vi "Simulate_RV_Core.vi"() -> ()   [LabVIEW 2011]
doc: "I. Description:\nThis example demonstrates how to continuously output a waveform using an internal sample clock. The automatic regeneration of data has been disabled, so new data has to be provided throughout the duration of the continuous Analog Output operation. This allows the generation of any arbitrary frequency as this VI computes new data for each iteration of the loop, maintaining phase continuity of the signal.\n\nII. Instructions for Running:\n1. Select the Physical Channel to correspond to where your signal is output on the DAQ device.\n2. Enter the Minimum and Maximum Voltage range.\n3. Specify the desired Sample Clock Rate of the output Waveform. Higher sample clock rates will produce a smoother waveform.\n4. Manually specify the Analog Output buffer size, in number of samples. A larger buffer would help non-regenerative operations avoid errors due to occasional high CPU load. \nNote: \nThe Analog Output buffer has to be at least as big as the amount of data being written to the board per iteration. The recommended buffer size would be at least twice the amount of data being written to the board per iteration.\n5. Enter the Waveform Information. See the documentation of the Basic Function Generator SubVI for information on each parameter.\n\nIII. Block Diagram Steps:\n1. Create an Analog Output Voltage channel.\n2. Configure the task to prohibit the automatic regeneration of data.\n3. Call the DAQmx (Sample Clock) VI to set the sample clock rate. Additionally, set the sample mode to Continuous.\n4. Read the actual sample clock rate (eventually coerced depending on the hardware used). \n5. Compute the desired waveform, using the buffer size and the actual update rate. This VI keeps track of the phase of the waveform to ensure that the generated signal is continuous.\n6. Write the waveform to the output buffer. \n7a. Call the Start VI. This is only needed when the loop is executed for the first time.\n7b. Do nothing.\n8. Loop continuously until user presses the Stop button. Every iteration computes and writes a new waveform to the buffer.\n9. Call the Clear Task VI to clear the Task.\n10. Use the popup dialog box to display an error or warning if any.\n\nIV. I/O Connections Overview:\nMake sure your signal output terminal matches the Physical Channel I/O Control. For further connection information, refer to your hardware reference manual."
uses:
  <vilib>/Utility/error.llb/DialogType.ctl
  <vilib>/DAQmx/write.llb/DAQmx Write (Analog 1D Wfm NChan NSamp).vi
  <vilib>/DAQmx/create/channels.llb/DAQmx Create Channel (AO-Voltage-Basic).vi
  <vilib>/DAQmx/configure/timing.llb/DAQmx Timing (Sample Clock).vi
  <vilib>/DAQmx/miscellaneous.llb/DAQmx Fill In Error Info.vi
  <vilib>/measure/NI_MABase.lvlib
  Program Files (x86)/National Instruments/LabVIEW 2011/resource/objmgr/daqmx.rc
panel:
  in  "Tab Control":T1(tab)=enum."RV"
  out "Trigger":waveform(dbl)(graph)={"t0"=timestamp(78.0 s since 1904-01-01), "dt"=0.0006666666666666666, "Y"=array[1200 elements]}
  in  "Trigg. level":sgl=2.0
  in  "Regular level":sgl=10.0
  in  "RV009_Ph":sgl[](array[numeric])=[0.0, 0.0, 0.0]
  in  "RV009_Amp":sgl[](array[numeric])=[0.9, 0.0, 0.0]
  in  "RV009.DC":sgl=5.0
  in  "RV008_Ph":sgl[](array[numeric])=[0.0, 0.0, 0.0]
  in  "RV008_Amp":sgl[](array[numeric])=[0.8, 0.0, 0.0]
  in  "RV008.DC":sgl=5.0
  in  "RV007_Ph":sgl[](array[numeric])=[0.0, 0.0, 0.0]
  in  "RV007_Amp":sgl[](array[numeric])=[0.4, 0.3, 0.4]
  in  "RV007.DC":sgl=5.0
  in  "RV006_Ph":sgl[](array[numeric])=[0.0, 0.0, 0.0]
  in  "RV006_Amp":sgl[](array[numeric])=[0.7, 0.3, 0.5]
  in  "RV006.DC":sgl=5.0
  out "RV":waveform(dbl)[](graph)=[{"t0"=timestamp(78.0 s since 1904-01-01), "dt"=0.0006666666666666666, "Y"=array[1200 elements]}, {"t0"=timestamp(78.0 s since 1904-01-01), "dt"=0.0006666666666666666, "Y"=array[1200 elements]}, {"t0"=timestamp(78.0 s since 1904-01-01), "dt"=0.0006666666666666666, "Y"=array[1200 elements]}, {"t0"=timestamp(78.0 s since 1904-01-01), "dt"=0.0006666666666666666, "Y"=array[1200 elements]}, {"t0"=timestamp(78.0 s since 1904-01-01), "dt"=0.0006666666666666666, "Y"=array[1200 elements]}, {"t0"=timestamp(78.0 s since 1904-01-01), "dt"=0.0006666666666666666, "Y"=array[1200 elements]}, {"t0"=timestamp(78.0 s since 1904-01-01), "dt"=0.0006666666666666666, "Y"=array[1200 elements]}, {"t0"=timestamp(78.0 s since 1904-01-01), "dt"=0.0006666666666666666, "Y"=array[1200 elements]}, {"t0"=timestamp(78.0 s since 1904-01-01), "dt"=0.0006666666666666666, "Y"=array[1200 elements]}, {"t0"=timestamp(78.0 s since 1904-01-01), "dt"=0.0006666666666666666, "Y"=array[1200 elements]}]
  in  "RV000_Ph":sgl[](array[numeric])=[0.0, 0.0, 0.0]
  in  "RV000_Amp":sgl[](array[numeric])=[0.4, 0.1, 0.3]
  in  "RV000.DC":sgl=5.0
  in  "RV001.DC":sgl=5.0
  in  "RV001_Amp":sgl[](array[numeric])=[0.8, 0.6, 0.2]
  in  "RV001_Ph":sgl[](array[numeric])=[90.0, 0.0, 0.0]
  in  "RV002_Ph":sgl[](array[numeric])=[0.0, 0.0, 0.0]
  in  "RV002_Amp":sgl[](array[numeric])=[0.3, 0.5, 0.3]
  in  "RV002.DC":sgl=5.0
  in  "RV003_Ph":sgl[](array[numeric])=[90.0, 0.0, 0.0]
  in  "RV003_Amp":sgl[](array[numeric])=[0.7, 0.4, 0.2]
  in  "RV003.DC":sgl=5.0
  in  "Multiplication factor":dbl=0.5
  in  "Add Noise":bool
  in  "RV004_Ph":sgl[](array[numeric])=[0.0, 0.0, 0.0]
  in  "RV004_Amp":sgl[](array[numeric])=[0.6, 0.3, 0.1]
  in  "RV004.DC":sgl=5.0
  in  "RV005_Ph":sgl[](array[numeric])=[0.0, 0.0, 0.0]
  in  "RV005_Amp":sgl[](array[numeric])=[0.9, 0.4, 0.2]
  in  "RV005.DC":sgl=5.0
  out "Proc1":waveform(dbl)(graph)={"t0"=timestamp(78.0 s since 1904-01-01), "dt"=0.0006666666666666666, "Y"=array[1200 elements]}
  in  "DC Proc Val 1":sgl=6.0
  out "Proc2":waveform(dbl)(graph)={"t0"=timestamp(78.0 s since 1904-01-01), "dt"=0.0006666666666666666, "Y"=array[1200 elements]}
  in  "DC Proc Val 2":sgl=1.0
  out "Loop Iteration":dbl=0.8050460815429688
  out "Waveform Graph":waveform(dbl)[](graph)=[{"t0"=timestamp(78.0 s since 1904-01-01), "dt"=0.0006666666666666666, "Y"=array[1200 elements]}, {"t0"=timestamp(78.0 s since 1904-01-01), "dt"=0.0006666666666666666, "Y"=array[1200 elements]}, {"t0"=timestamp(78.0 s since 1904-01-01), "dt"=0.0006666666666666666, "Y"=array[1200 elements]}, {"t0"=timestamp(78.0 s since 1904-01-01), "dt"=0.0006666666666666666, "Y"=array[1200 elements]}, {"t0"=timestamp(78.0 s since 1904-01-01), "dt"=0.0006666666666666666, "Y"=array[1200 elements]}, {"t0"=timestamp(78.0 s since 1904-01-01), "dt"=0.0006666666666666666, "Y"=array[1200 elements]}, {"t0"=timestamp(78.0 s since 1904-01-01), "dt"=0.0006666666666666666, "Y"=array[1200 elements]}, {"t0"=timestamp(78.0 s since 1904-01-01), "dt"=0.0006666666666666666, "Y"=array[1200 elements]}, {"t0"=timestamp(78.0 s since 1904-01-01), "dt"=0.0006666666666666666, "Y"=array[1200 elements]}, {"t0"=timestamp(78.0 s since 1904-01-01), "dt"=0.0006666666666666666, "Y"=array[1200 elements]}, {"t0"=timestamp(78.0 s since 1904-01-01), "dt"=0.0006666666666666666, "Y"=array[1200 elements]}, {"t0"=timestamp(78.0 s since 1904-01-01), "dt"=0.0006666666666666666, "Y"=array[1200 elements]}, {"t0"=timestamp(78.0 s since 1904-01-01), "dt"=0.0006666666666666666, "Y"=array[1200 elements]}] caption="Output Waveforms"
  in  "stop":bool
  # "s"
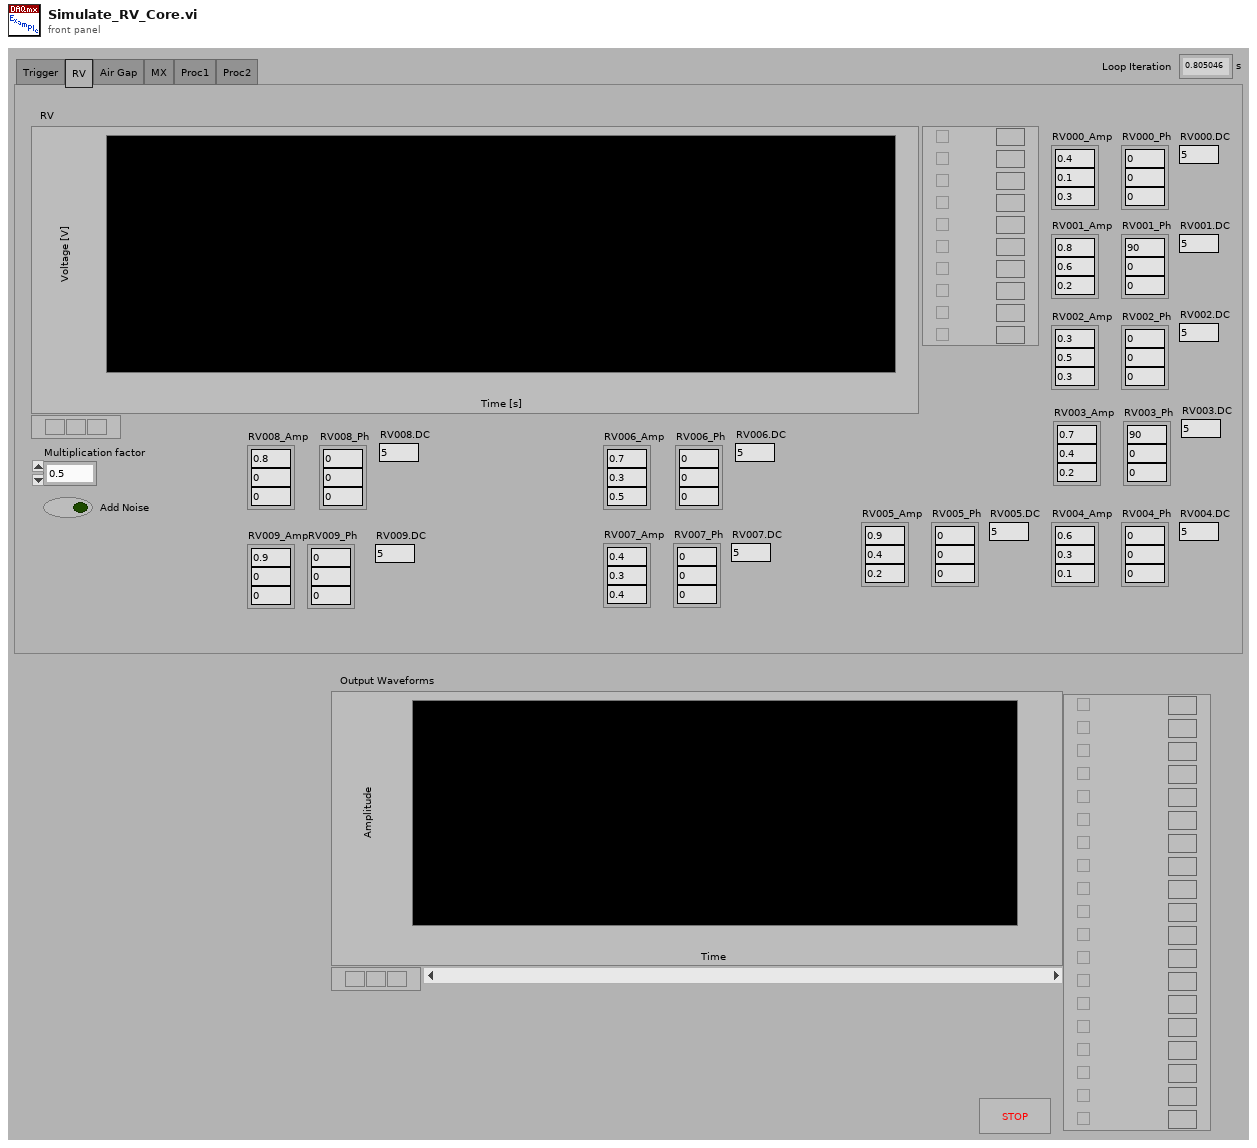
[diagram p1: front panel]
types:
  T1 = enum32{"Trigger", "RV", "Air Gap", "MX", "Proc1", "Proc2"}
  T2 = typedef "DialogType.ctl" = u16
  T3 = enum16{"Sine Wave", "Triangle Wave", "Square Wave", "Sawtooth Wave"}
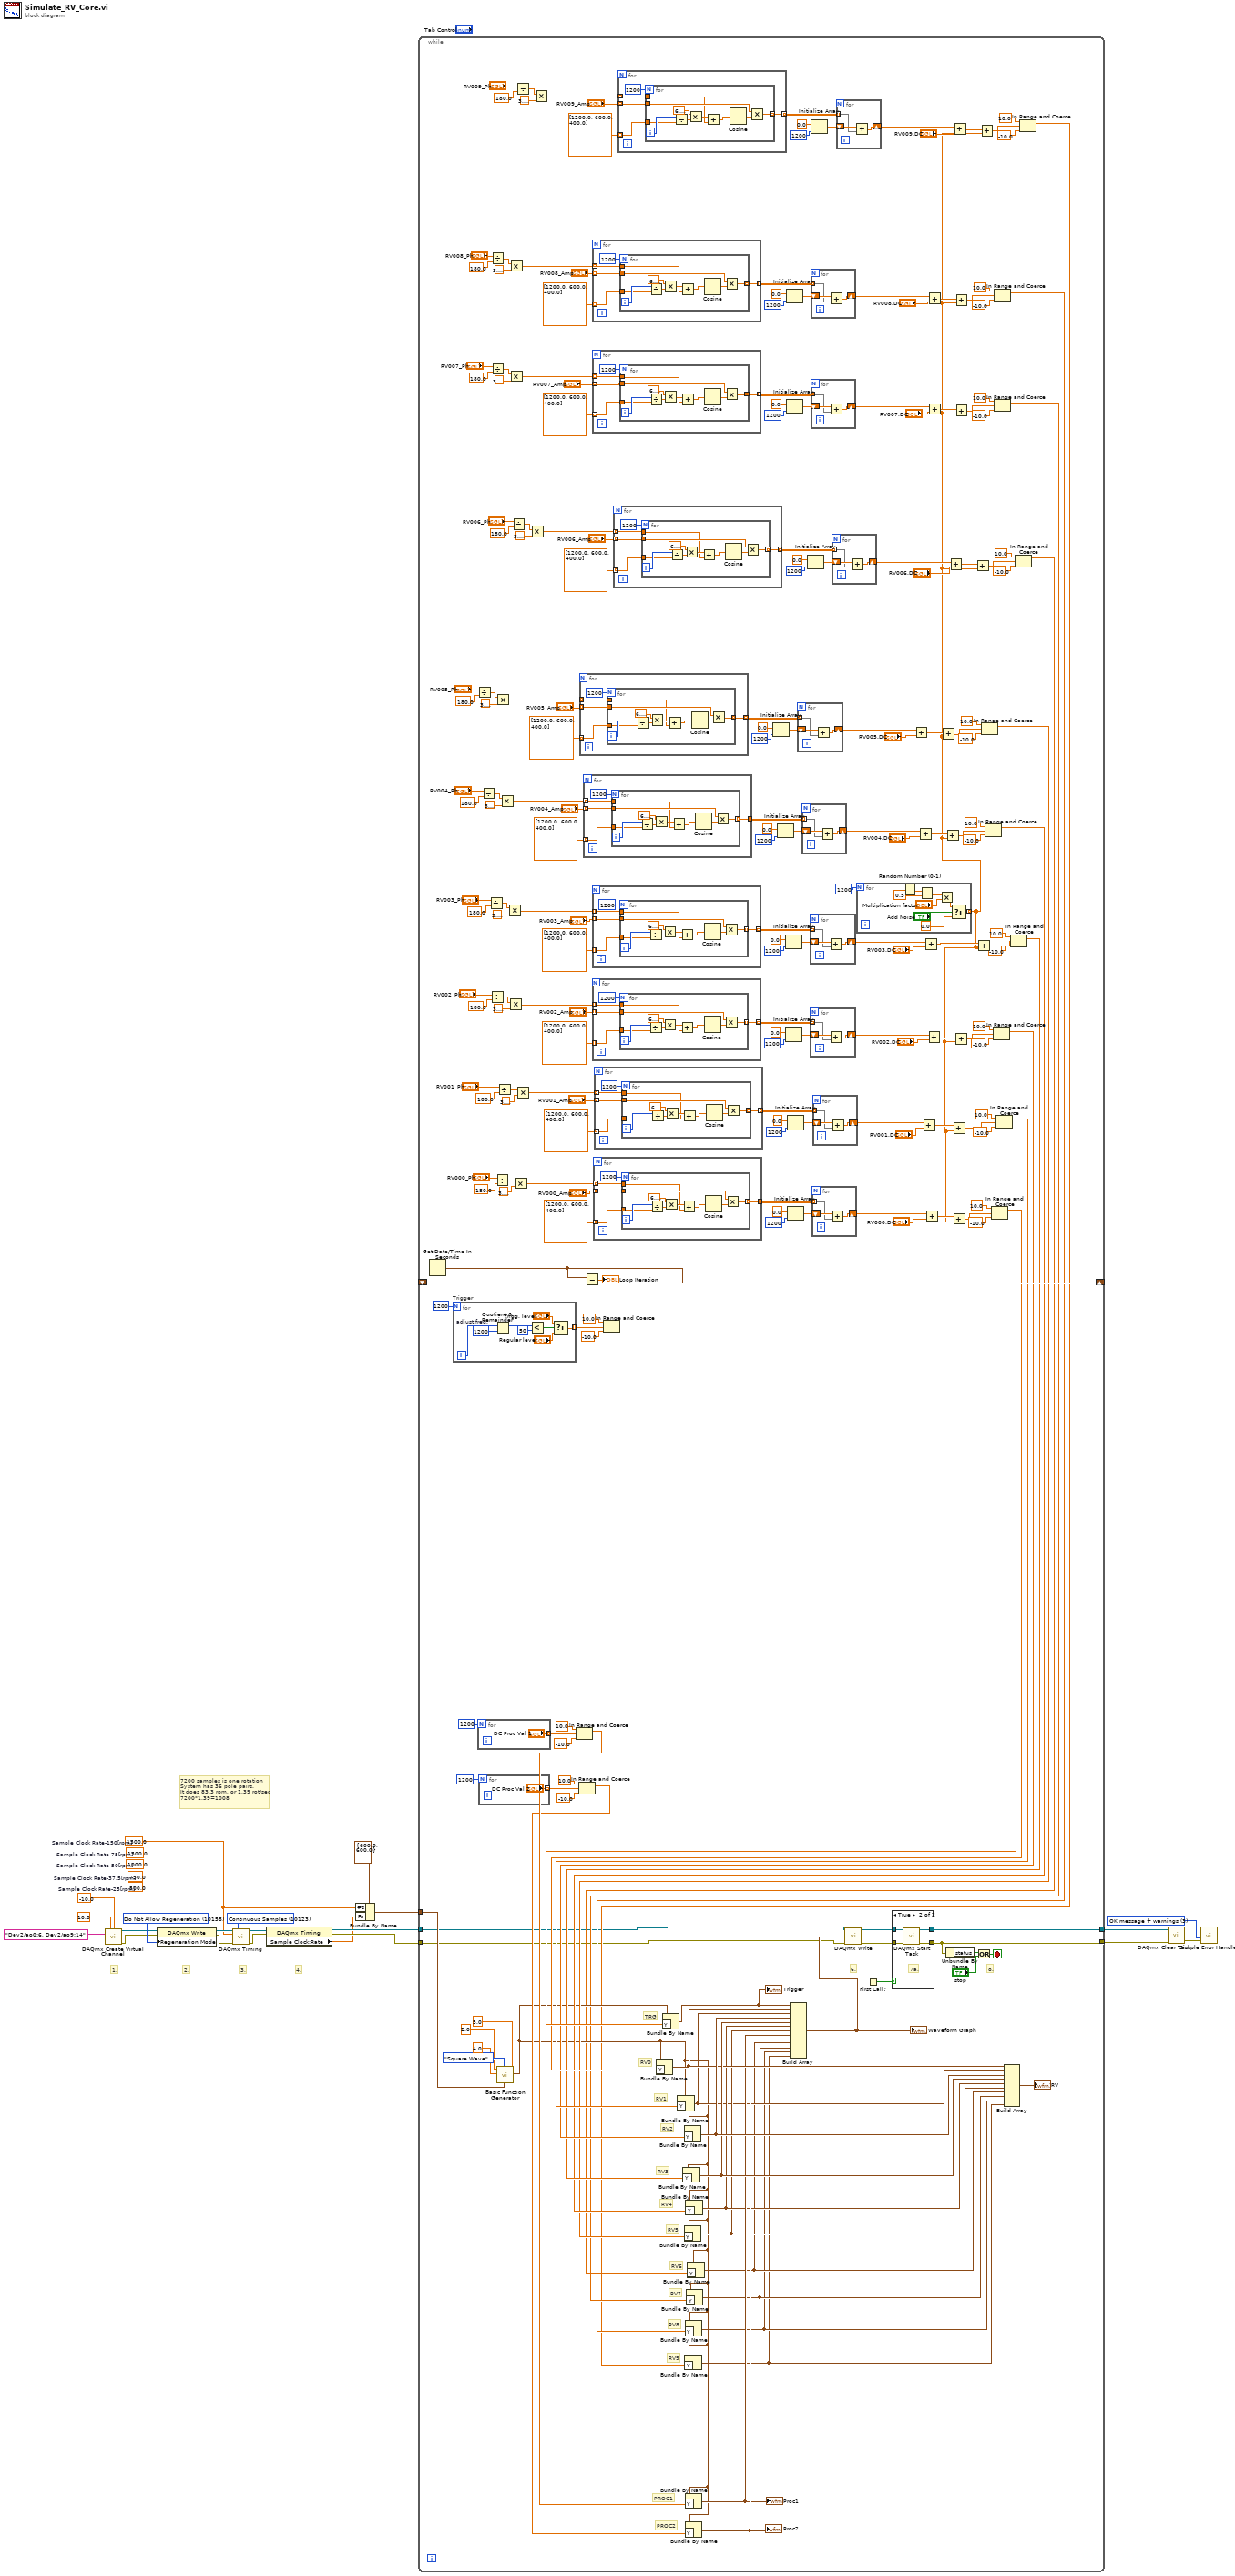
[diagram p0: block diagram]
diagram:
  w1 = 1500.0  # Sample Clock Rate-150[rpm]
  (unwired) 1000.0  # Sample Clock Rate-50[rpm]
  (unwired) 500.0  # Sample Clock Rate-25[rpm]
  (unwired) 750.0  # Sample Clock Rate-37.5[rpm]
  (unwired) 1500.0  # Sample Clock Rate-75[rpm]
  w11 = 10158 items=["Allow Regeneration"=10097, "Do Not Allow Regeneration"=10158] ("RegenMode")
  w17 = T2 3 items=["no dialog", "OK message", "continue or stop message", "OK message + warnings", "continue/stop + warnings"] ("type of dialog (OK msg:1)")
  w20 = 10123 items=["Finite Samples"=10178, "Continuous Samples"=10123] ("sample mode")
  # "7200 samples is one rotation\nSystem has 36 pole pairs.\nIt does 83.3 rpm, or 1.39 rot/sec\n7200*1.39=1008"
  # "4."
  # "3."
  # "2."
  # "1."
  n1 = call-poly <vilib>:"DAQmx Create Virtual Channel.vi"("maximum value"=10.0 ("Maximum Value"), "minimum value"=-10.0 ("Minimum Value"), "physical channels"=tag "Dev2/ao0:6, Dev2/ao9:14" ("Physical Channels")) -> ("task out"=w10:refnum<k21>, "error out"=w9:errorcluster)  [unwired: 6 in, 5 out]
  n2 = property class="DAQmx Write"(reference=w10, error in=w9, "Regeneration Mode"=w11) -> (reference out=w6:refnum<k21>, error out=w5:errorcluster)
  n3 = call-poly <vilib>:"DAQmx Timing.vi"("task/channels in"=w6, "sample mode"=w20, "rate"=w1, "error in"=w5) -> ("task out"=w3:refnum<k21>, "error out"=w14:errorcluster)  [unwired: 3 in, 7 out]
  n4 = property class="DAQmx Timing"(reference=w3, error in=w14) -> (reference out=w8:refnum<k21>, error out=w7:errorcluster, "Sample Clock:Rate"=w4:dbl)
  n5 = Bundle By Name(cluster=cluster{"Fs":dbl, "#s":dbl} {"Fs"=600.0, "#s"=600.0} ("sampling info"), "#s"=w1, "Fs"=w4) -> (w12:cluster{"Fs":dbl, "#s":dbl})
  n6 = while {
    tunnel: w8 -> [w23]
    tunnel: [w246] -> w16
    tunnel: w7 -> [w22]
    tunnel: [w247] -> w15
    tunnel: w12 -> [w238]
    shift-right: [w244] -> _
    shift-left: _ -> [w233]
    stop <- w252 stop-if-true
    # "RV9"
    # "RV8"
    # "RV7"
    # "RV6"
    # "PROC2"
    # "PROC1"
    # "RV5"
    # "RV4"
    # "RV3"
    # "RV2"
    # "RV1"
    # "TRG"
    # "RV0"
    # "8."
    # "6."
    n7 = Get Date/Time In Seconds() -> (seconds since 1Jan1904=w244:timestamp)
    n8 = for "Trigger" {
      N: 1200 -> [_]
      tunnel: [w444] -> w230 mode=indexing
      i -> [w450]
      w449 = 1200  # adjust freq.
      n9 = Quotient & Remainder(x=w450, y=w449) -> (x-y*floor(x/y)=w448:i32)  [unwired: 1 out]
      n10 = Less?(x=w448, y=50) -> (x < y?=w443:bool)
      n11 = Select(t="Trigg. level", s=w443, f="Regular level") -> (s? t:f=w444:sgl)
    }
    n12 = Divide(x="RV005_Ph", y=sgl 180.0) -> (x/y=w113:sgl[])
    n13 = for {
      N: 1200 -> [_]
      tunnel: ["DC Proc Val 1"] -> w159 mode=indexing
    }
    n14 = for {
      N: 1200 -> [_]
      tunnel: ["DC Proc Val 2"] -> w155 mode=indexing
    }
    n15 = Divide(x="RV004_Ph", y=sgl 180.0) -> (x/y=w130:sgl[])
    n16 = Divide(x="RV003_Ph", y=sgl 180.0) -> (x/y=w164:sgl[])
    n17 = Divide(x="RV002_Ph", y=sgl 180.0) -> (x/y=w168:sgl[])
    n18 = Divide(x="RV008_Ph", y=sgl 180.0) -> (x/y=w63:sgl[])
    n19 = Divide(x="RV007_Ph", y=sgl 180.0) -> (x/y=w77:sgl[])
    n20 = Divide(x="RV000_Ph", y=sgl 180.0) -> (x/y=w179:sgl[])
    n21 = Multiply(x=w113, y=sgl 3.1415927) -> (x*y=w112:sgl[])
    n22 = Divide(x="RV001_Ph", y=sgl 180.0) -> (x/y=w173:sgl[])
    n23 = call <vilib>:"Basic Function Generator.vi"("offset"=5.0 ("offset 5"), "sampling info"=w238, "signal type"=T3."Square Wave" ("Waveform Type 5"), "amplitude"=4.0 ("Amplitude 5"), "frequency"=2.0 ("Frequency 5")) -> ("signal out"=w33:waveform(dbl))  [unwired: 4 in, 2 out]
    n24 = Multiply(x=w130, y=sgl 3.1415927) -> (x*y=w129:sgl[])
    n25 = Multiply(x=w164, y=sgl 3.1415927) -> (x*y=w162:sgl[])
    n26 = Multiply(x=w168, y=sgl 3.1415927) -> (x*y=w167:sgl[])
    n27 = Multiply(x=w63, y=sgl 3.1415927) -> (x*y=w62:sgl[])
    n28 = Multiply(x=w77, y=sgl 3.1415927) -> (x*y=w76:sgl[])
    n29 = Divide(x="RV006_Ph", y=sgl 180.0) -> (x/y=w91:sgl[])
    n30 = Multiply(x=w179, y=sgl 3.1415927) -> (x*y=w177:sgl[])
    n31 = Divide(x="RV009_Ph", y=sgl 180.0) -> (x/y=w49:sgl[])
    n32 = Multiply(x=w173, y=sgl 3.1415927) -> (x*y=w172:sgl[])
    n33 = Multiply(x=w91, y=sgl 3.1415927) -> (x*y=w90:sgl[])
    n34 = Multiply(x=w49, y=sgl 3.1415927) -> (x*y=w48:sgl[])
    n35 = In Range and Coerce(upper limit=sgl 10.0, x=w159, lower limit=sgl -10.0) -> (coerced(x)=w158:sgl[])  [unwired: 1 out]
    n36 = In Range and Coerce(upper limit=sgl 10.0, x=w155, lower limit=sgl -10.0) -> (coerced(x)=w154:sgl[])  [unwired: 1 out]
    n37 = for {
      tunnel: w112 -> [w331] mode=indexing
      tunnel: "RV005_Amp" -> [w330] mode=indexing
      tunnel: sgl[] [1200.0, 600.0, 400.0] -> [w329] mode=indexing
      tunnel: [w328] -> w120 mode=indexing
      n38 = for {
        N: 1200 -> [_]
        tunnel: w330 -> [w338]
        tunnel: [w337] -> w328 mode=indexing
        tunnel: w331 -> [w334]
        tunnel: w329 -> [w333]
        i -> [w342]
        n39 = Divide(x=w342, y=w333) -> (x/y=w341:sgl)
        n40 = Multiply(x=sgl 6.2831855, y=w341) -> (x*y=w336:sgl)
        n41 = Add(x=w336, y=w334) -> (x+y=w335:sgl)
        n42 = Cosine(x=w335) -> (cos(x)=w339:sgl)
        n43 = Multiply(x=w338, y=w339) -> (x*y=w337:sgl)
      }
    }
    n44 = for {
      tunnel: w129 -> [w349] mode=indexing
      tunnel: "RV004_Amp" -> [w348] mode=indexing
      tunnel: sgl[] [1200.0, 600.0, 400.0] -> [w347] mode=indexing
      tunnel: [w346] -> w137 mode=indexing
      n45 = for {
        N: 1200 -> [_]
        tunnel: w348 -> [w356]
        tunnel: [w355] -> w346 mode=indexing
        tunnel: w349 -> [w352]
        tunnel: w347 -> [w351]
        i -> [w360]
        n46 = Divide(x=w360, y=w351) -> (x/y=w359:sgl)
        n47 = Multiply(x=sgl 6.2831855, y=w359) -> (x*y=w354:sgl)
        n48 = Add(x=w354, y=w352) -> (x+y=w353:sgl)
        n49 = Cosine(x=w353) -> (cos(x)=w357:sgl)
        n50 = Multiply(x=w356, y=w357) -> (x*y=w355:sgl)
      }
    }
    n51 = Subtract(x=w244, y=w233) -> (x-y=→"Loop Iteration":dbl)
    n52 = for {
      tunnel: w162 -> [w375] mode=indexing
      tunnel: "RV003_Amp" -> [w374] mode=indexing
      tunnel: sgl[] [1200.0, 600.0, 400.0] -> [w373] mode=indexing
      tunnel: [w372] -> w198 mode=indexing
      n53 = for {
        N: 1200 -> [_]
        tunnel: w374 -> [w382]
        tunnel: [w381] -> w372 mode=indexing
        tunnel: w375 -> [w378]
        tunnel: w373 -> [w377]
        i -> [w386]
        n54 = Divide(x=w386, y=w377) -> (x/y=w385:sgl)
        n55 = Multiply(x=sgl 6.2831855, y=w385) -> (x*y=w380:sgl)
        n56 = Add(x=w380, y=w378) -> (x+y=w379:sgl)
        n57 = Cosine(x=w379) -> (cos(x)=w383:sgl)
        n58 = Multiply(x=w382, y=w383) -> (x*y=w381:sgl)
      }
    }
    n59 = for {
      tunnel: w167 -> [w393] mode=indexing
      tunnel: "RV002_Amp" -> [w392] mode=indexing
      tunnel: sgl[] [1200.0, 600.0, 400.0] -> [w391] mode=indexing
      tunnel: [w390] -> w201 mode=indexing
      n60 = for {
        N: 1200 -> [_]
        tunnel: w392 -> [w400]
        tunnel: [w399] -> w390 mode=indexing
        tunnel: w393 -> [w396]
        tunnel: w391 -> [w395]
        i -> [w404]
        n61 = Divide(x=w404, y=w395) -> (x/y=w403:sgl)
        n62 = Multiply(x=sgl 6.2831855, y=w403) -> (x*y=w398:sgl)
        n63 = Add(x=w398, y=w396) -> (x+y=w397:sgl)
        n64 = Cosine(x=w397) -> (cos(x)=w401:sgl)
        n65 = Multiply(x=w400, y=w401) -> (x*y=w399:sgl)
      }
    }
    n66 = for {
      tunnel: w62 -> [w277] mode=indexing
      tunnel: "RV008_Amp" -> [w276] mode=indexing
      tunnel: sgl[] [1200.0, 600.0, 400.0] -> [w275] mode=indexing
      tunnel: [w274] -> w67 mode=indexing
      n67 = for {
        N: 1200 -> [_]
        tunnel: w276 -> [w284]
        tunnel: [w283] -> w274 mode=indexing
        tunnel: w277 -> [w280]
        tunnel: w275 -> [w279]
        i -> [w288]
        n68 = Divide(x=w288, y=w279) -> (x/y=w287:sgl)
        n69 = Multiply(x=sgl 6.2831855, y=w287) -> (x*y=w282:sgl)
        n70 = Add(x=w282, y=w280) -> (x+y=w281:sgl)
        n71 = Cosine(x=w281) -> (cos(x)=w285:sgl)
        n72 = Multiply(x=w284, y=w285) -> (x*y=w283:sgl)
      }
    }
    n73 = for {
      tunnel: w76 -> [w295] mode=indexing
      tunnel: sgl[] [1200.0, 600.0, 400.0] -> [w294] mode=indexing
      tunnel: [w293] -> w81 mode=indexing
      tunnel: "RV007_Amp" -> [w292] mode=indexing
      n74 = for {
        N: 1200 -> [_]
        tunnel: w292 -> [w302]
        tunnel: [w301] -> w293 mode=indexing
        tunnel: w295 -> [w298]
        tunnel: w294 -> [w297]
        i -> [w306]
        n75 = Divide(x=w306, y=w297) -> (x/y=w305:sgl)
        n76 = Multiply(x=sgl 6.2831855, y=w305) -> (x*y=w300:sgl)
        n77 = Add(x=w300, y=w298) -> (x+y=w299:sgl)
        n78 = Cosine(x=w299) -> (cos(x)=w303:sgl)
        n79 = Multiply(x=w302, y=w303) -> (x*y=w301:sgl)
      }
    }
    n80 = for {
      tunnel: w177 -> [w429] mode=indexing
      tunnel: "RV000_Amp" -> [w428] mode=indexing
      tunnel: sgl[] [1200.0, 600.0, 400.0] -> [w427] mode=indexing
      tunnel: [w426] -> w225 mode=indexing
      n81 = for {
        N: 1200 -> [_]
        tunnel: w428 -> [w436]
        tunnel: [w435] -> w426 mode=indexing
        tunnel: w429 -> [w432]
        tunnel: w427 -> [w431]
        i -> [w440]
        n82 = Divide(x=w440, y=w431) -> (x/y=w439:sgl)
        n83 = Multiply(x=sgl 6.2831855, y=w439) -> (x*y=w434:sgl)
        n84 = Add(x=w434, y=w432) -> (x+y=w433:sgl)
        n85 = Cosine(x=w433) -> (cos(x)=w437:sgl)
        n86 = Multiply(x=w436, y=w437) -> (x*y=w435:sgl)
      }
    }
    n87 = for {
      tunnel: w172 -> [w411] mode=indexing
      tunnel: "RV001_Amp" -> [w410] mode=indexing
      tunnel: sgl[] [1200.0, 600.0, 400.0] -> [w409] mode=indexing
      tunnel: [w408] -> w216 mode=indexing
      n88 = for {
        N: 1200 -> [_]
        tunnel: w410 -> [w418]
        tunnel: [w417] -> w408 mode=indexing
        tunnel: w411 -> [w414]
        tunnel: w409 -> [w413]
        i -> [w422]
        n89 = Divide(x=w422, y=w413) -> (x/y=w421:sgl)
        n90 = Multiply(x=sgl 6.2831855, y=w421) -> (x*y=w416:sgl)
        n91 = Add(x=w416, y=w414) -> (x+y=w415:sgl)
        n92 = Cosine(x=w415) -> (cos(x)=w419:sgl)
        n93 = Multiply(x=w418, y=w419) -> (x*y=w417:sgl)
      }
    }
    n94 = In Range and Coerce(upper limit=sgl 10.0, x=w230, lower limit=sgl -10.0) -> (coerced(x)=w229:sgl[])  [unwired: 1 out]
    n95 = for {
      tunnel: w90 -> [w313] mode=indexing
      tunnel: "RV006_Amp" -> [w312] mode=indexing
      tunnel: sgl[] [1200.0, 600.0, 400.0] -> [w311] mode=indexing
      tunnel: [w310] -> w95 mode=indexing
      n96 = for {
        N: 1200 -> [_]
        tunnel: w312 -> [w320]
        tunnel: [w319] -> w310 mode=indexing
        tunnel: w313 -> [w316]
        tunnel: w311 -> [w315]
        i -> [w324]
        n97 = Divide(x=w324, y=w315) -> (x/y=w323:sgl)
        n98 = Multiply(x=sgl 6.2831855, y=w323) -> (x*y=w318:sgl)
        n99 = Add(x=w318, y=w316) -> (x+y=w317:sgl)
        n100 = Cosine(x=w317) -> (cos(x)=w321:sgl)
        n101 = Multiply(x=w320, y=w321) -> (x*y=w319:sgl)
      }
    }
    n102 = for {
      tunnel: w48 -> [w259] mode=indexing
      tunnel: "RV009_Amp" -> [w258] mode=indexing
      tunnel: sgl[] [1200.0, 600.0, 400.0] -> [w257] mode=indexing
      tunnel: [w256] -> w53 mode=indexing
      n103 = for {
        N: 1200 -> [_]
        tunnel: w258 -> [w266]
        tunnel: [w265] -> w256 mode=indexing
        tunnel: w259 -> [w262]
        tunnel: w257 -> [w261]
        i -> [w270]
        n104 = Divide(x=w270, y=w261) -> (x/y=w269:sgl)
        n105 = Multiply(x=sgl 6.2831855, y=w269) -> (x*y=w264:sgl)
        n106 = Add(x=w264, y=w262) -> (x+y=w263:sgl)
        n107 = Cosine(x=w263) -> (cos(x)=w267:sgl)
        n108 = Multiply(x=w266, y=w267) -> (x*y=w265:sgl)
      }
    }
    n109 = Bundle By Name(cluster=w33, "Y"=w229) -> (w103:waveform(dbl))
    "Trigger" <- w103
    n110 = Bundle By Name(cluster=w33, "Y"=w158) -> (w108:waveform(dbl))
    "Proc1" <- w108
    n111 = Bundle By Name(cluster=w33, "Y"=w154) -> (w109:waveform(dbl))
    "Proc2" <- w109
    n112 = Initialize Array(sgl 0.0, 1200 ("dimension size")) -> (w124:sgl[])
    n113 = Initialize Array(sgl 0.0, 1200 ("dimension size")) -> (w141:sgl[])
    n114 = Initialize Array(sgl 0.0, 1200 ("dimension size")) -> (w194:sgl[])
    n115 = Initialize Array(sgl 0.0, 1200 ("dimension size")) -> (w205:sgl[])
    n116 = Initialize Array(sgl 0.0, 1200 ("dimension size")) -> (w71:sgl[])
    n117 = Initialize Array(sgl 0.0, 1200 ("dimension size")) -> (w85:sgl[])
    n118 = Initialize Array(sgl 0.0, 1200 ("dimension size")) -> (w220:sgl[])
    n119 = Initialize Array(sgl 0.0, 1200 ("dimension size")) -> (w212:sgl[])
    n120 = for {
      shift-right: [w325] -> w118
      shift-left: w124 -> [w327]
      tunnel: w120 -> [w326] mode=indexing
      n121 = Add(x=w327, y=w326) -> (x+y=w325:sgl[])
    }
    n122 = for {
      shift-right: [w343] -> w135
      shift-left: w141 -> [w345]
      tunnel: w137 -> [w344] mode=indexing
      n123 = Add(x=w345, y=w344) -> (x+y=w343:sgl[])
    }
    n124 = Initialize Array(sgl 0.0, 1200 ("dimension size")) -> (w99:sgl[])
    n125 = for {
      shift-right: [w369] -> w183
      shift-left: w194 -> [w371]
      tunnel: w198 -> [w370] mode=indexing
      n126 = Add(x=w371, y=w370) -> (x+y=w369:sgl[])
    }
    n127 = for {
      shift-right: [w387] -> w185
      shift-left: w205 -> [w389]
      tunnel: w201 -> [w388] mode=indexing
      n128 = Add(x=w389, y=w388) -> (x+y=w387:sgl[])
    }
    n129 = for {
      shift-right: [w271] -> w66
      shift-left: w71 -> [w273]
      tunnel: w67 -> [w272] mode=indexing
      n130 = Add(x=w273, y=w272) -> (x+y=w271:sgl[])
    }
    n131 = for {
      shift-right: [w289] -> w80
      shift-left: w85 -> [w291]
      tunnel: w81 -> [w290] mode=indexing
      n132 = Add(x=w291, y=w290) -> (x+y=w289:sgl[])
    }
    n133 = Initialize Array(sgl 0.0, 1200 ("dimension size")) -> (w57:sgl[])
    n134 = for {
      shift-right: [w423] -> w189
      shift-left: w220 -> [w425]
      tunnel: w225 -> [w424] mode=indexing
      n135 = Add(x=w425, y=w424) -> (x+y=w423:sgl[])
    }
    n136 = for {
      shift-right: [w405] -> w187
      shift-left: w212 -> [w407]
      tunnel: w216 -> [w406] mode=indexing
      n137 = Add(x=w407, y=w406) -> (x+y=w405:sgl[])
    }
    n138 = for {
      shift-right: [w307] -> w94
      shift-left: w99 -> [w309]
      tunnel: w95 -> [w308] mode=indexing
      n139 = Add(x=w309, y=w308) -> (x+y=w307:sgl[])
    }
    n140 = for {
      shift-right: [w253] -> w52
      shift-left: w57 -> [w255]
      tunnel: w53 -> [w254] mode=indexing
      n141 = Add(x=w255, y=w254) -> (x+y=w253:sgl[])
    }
    n142 = for {
      N: 1200 -> [_]
      tunnel: [w361] -> w30 mode=indexing
      n143 = Random Number (0-1)() -> (number: 0 to 1=w366:dbl)
      n144 = Subtract(x=w366, y=0.5) -> (x-y=w364:dbl)
      n145 = Multiply(x=w364, y="Multiplication factor") -> (x*y=w362:dbl)
      n146 = Select(t=w362, s="Add Noise", f=0.0) -> (s? t:f=w361:dbl)
    }
    n147 = First Call?() -> (First Call?: T/F=w245:bool)
    n148 = Add(x=w118, y="RV005.DC") -> (x+y=w111:sgl[])
    n149 = Add(x=w135, y="RV004.DC") -> (x+y=w128:sgl[])
    n150 = Add(x=w187, y="RV001.DC") -> (x+y=w148:sgl[])
    n151 = Add(x=w183, y="RV003.DC") -> (x+y=w152:sgl[])
    n152 = Add(x=w189, y="RV000.DC") -> (x+y=w146:sgl[])
    n153 = Add(x=w185, y="RV002.DC") -> (x+y=w150:sgl[])
    n154 = Add(x=w66, y="RV008.DC") -> (x+y=w61:sgl[])
    n155 = Add(x=w80, y="RV007.DC") -> (x+y=w75:sgl[])
    n156 = Add(x=w111, y=w30) -> (x+y=w110:dbl[])
    n157 = Add(x=w128, y=w30) -> (x+y=w127:dbl[])
    n158 = Add(x=w94, y="RV006.DC") -> (x+y=w89:sgl[])
    n159 = Add(x=w148, y=w30) -> (x+y=w147:dbl[])
    n160 = Add(x=w146, y=w30) -> (x+y=w145:dbl[])
    n161 = Add(x=w52, y="RV009.DC") -> (x+y=w47:sgl[])
    n162 = Add(x=w150, y=w30) -> (x+y=w149:dbl[])
    n163 = Add(x=w61, y=w30) -> (x+y=w60:dbl[])
    n164 = Add(x=w75, y=w30) -> (x+y=w74:dbl[])
    n165 = Add(x=w89, y=w30) -> (x+y=w88:dbl[])
    n166 = Add(x=w152, y=w30) -> (x+y=w151:dbl[])
    n167 = Add(x=w47, y=w30) -> (x+y=w46:dbl[])
    n168 = In Range and Coerce(upper limit=sgl 10.0, x=w110, lower limit=sgl -10.0) -> (coerced(x)=w106:dbl[])  [unwired: 1 out]
    n169 = Bundle By Name(cluster=w33, "Y"=w106) -> (w104:waveform(dbl))
    n170 = In Range and Coerce(upper limit=sgl 10.0, x=w127, lower limit=sgl -10.0) -> (coerced(x)=w107:dbl[])  [unwired: 1 out]
    n171 = Bundle By Name(cluster=w33, "Y"=w107) -> (w105:waveform(dbl))
    n172 = In Range and Coerce(upper limit=sgl 10.0, x=w145, lower limit=sgl -10.0) -> (coerced(x)=w217:dbl[])  [unwired: 1 out]
    n173 = Bundle By Name(cluster=w33, "Y"=w217) -> (w144:waveform(dbl))
    n174 = In Range and Coerce(upper limit=sgl 10.0, x=w149, lower limit=sgl -10.0) -> (coerced(x)=w199:dbl[])  [unwired: 1 out]
    n175 = Bundle By Name(cluster=w33, "Y"=w199) -> (w228:waveform(dbl))
    n176 = In Range and Coerce(upper limit=sgl 10.0, x=w60, lower limit=sgl -10.0) -> (coerced(x)=w29:dbl[])  [unwired: 1 out]
    n177 = Bundle By Name(cluster=w33, "Y"=w29) -> (w25:waveform(dbl))
    n178 = In Range and Coerce(upper limit=sgl 10.0, x=w74, lower limit=sgl -10.0) -> (coerced(x)=w31:dbl[])  [unwired: 1 out]
    n179 = Bundle By Name(cluster=w33, "Y"=w31) -> (w26:waveform(dbl))
    n180 = In Range and Coerce(upper limit=sgl 10.0, x=w147, lower limit=sgl -10.0) -> (coerced(x)=w208:dbl[])  [unwired: 1 out]
    n181 = Bundle By Name(cluster=w33, "Y"=w208) -> (w102:waveform(dbl))
    n182 = In Range and Coerce(upper limit=sgl 10.0, x=w151, lower limit=sgl -10.0) -> (coerced(x)=w190:dbl[])  [unwired: 1 out]
    n183 = Bundle By Name(cluster=w33, "Y"=w190) -> (w227:waveform(dbl))
    n184 = In Range and Coerce(upper limit=sgl 10.0, x=w88, lower limit=sgl -10.0) -> (coerced(x)=w32:dbl[])  [unwired: 1 out]
    n185 = Bundle By Name(cluster=w33, "Y"=w32) -> (w27:waveform(dbl))
    n186 = In Range and Coerce(upper limit=sgl 10.0, x=w46, lower limit=sgl -10.0) -> (coerced(x)=w28:dbl[])  [unwired: 1 out]
    n187 = Bundle By Name(cluster=w33, "Y"=w28) -> (w24:waveform(dbl))
    n188 = Build Array(w103, w144, w102, w228, w227, w105, w104, w108, w109, w27, w26, w25, w24) -> (w237:waveform(dbl)[])
    "Waveform Graph" <- w237
    n189 = call-poly <vilib>:"DAQmx Write.vi"("task/channels in"=w23, "data"=w237, "error in"=w22) -> ("task out"=w249:refnum<k21>, "error out"=w248:errorcluster)  [unwired: 1 in, 10 out]
    n190 = case shown="True" w245 {
      tunnel: w249 -> [w452 w456]
      tunnel: w248 -> [w451 w455]
      tunnel: [w451 w454] -> w247
      tunnel: [w452 w453] -> w246
      frame False {
        # "7b."
      }
      frame True {
        # "7a."
        n191 = call <vilib>:"DAQmx Start Task.vi"("task/channels in"=w456, "error in"=w455) -> ("task out"=w453:refnum<k21>, "error out"=w454:errorcluster)  [unwired: 12 out]
      }
    }
    n192 = Unbundle By Name(w247) -> ("status"=w251:bool)
    n193 = Or(x=w251, y="stop") -> (x .or. y?=w252:bool)
    n194 = Build Array(w144, w102, w228, w227, w105, w104, w27, w26, w25, w24) -> (→"RV":waveform(dbl)[])
  }
  n195 = call <vilib>:"DAQmx Clear Task.vi"("task in"=w16, "error in"=w15) -> ("error out"=w21:errorcluster)  [unwired: 13 out]
  n196 = call <vilib>:"Simple Error Handler.vi"("type of dialog (OK msg:1)"=w17, "error in (no error)"=w21) -> ()  [unwired: 8 out]
